vi "advance array manipulation part3.vi"() -> ()   [LabVIEW 2016]
panel:
  in  "Rotate index":i32
  out "Rotated Array":dbl[](array[numeric])
  in  "1D Input Array":dbl[](array[numeric])
  out "Reversed Array":dbl[](array[numeric])
  in  "1D Input Array":dbl[](array[numeric])
  out "Splited second Array":dbl[](array[numeric])
  out "Splited first Array":dbl[](array[numeric])
  in  "Split index":i32
  in  "1D Input Array":dbl[](array[numeric])
  out "Output index":i32
  in  "Search index":i32
  in  "Element":dbl
  in  "1D Input Array":dbl[](array[numeric])
  out "Output Array":dbl[](array[numeric])
  in  "1D Input Array":dbl[](array[numeric])
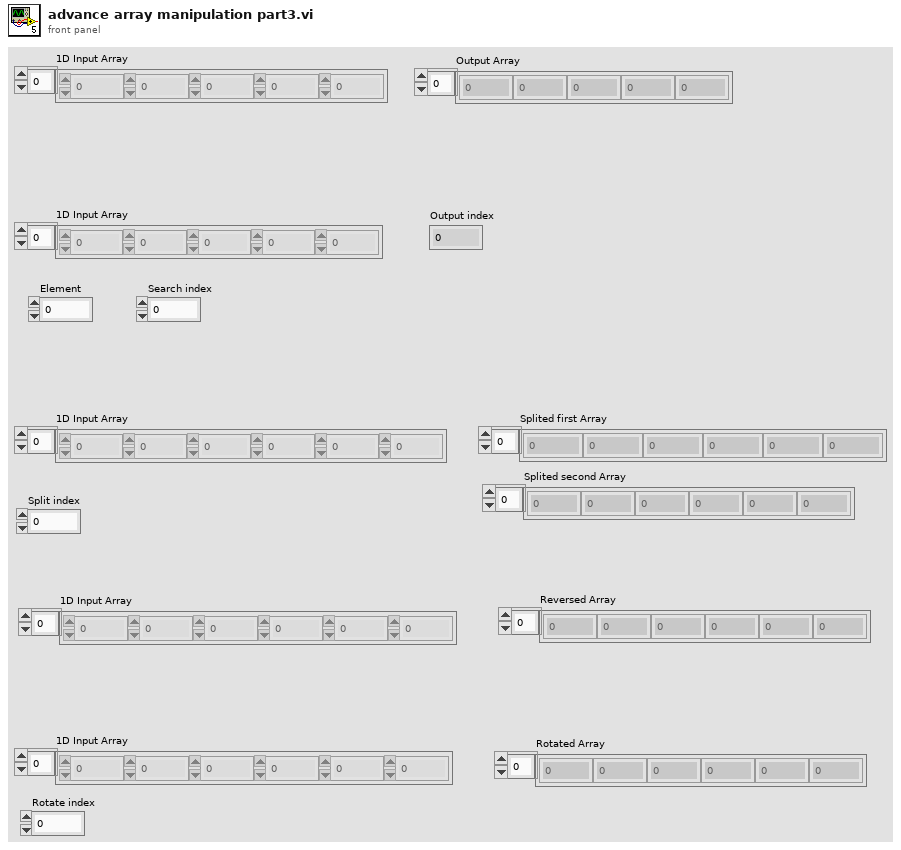
[diagram p1: front panel]
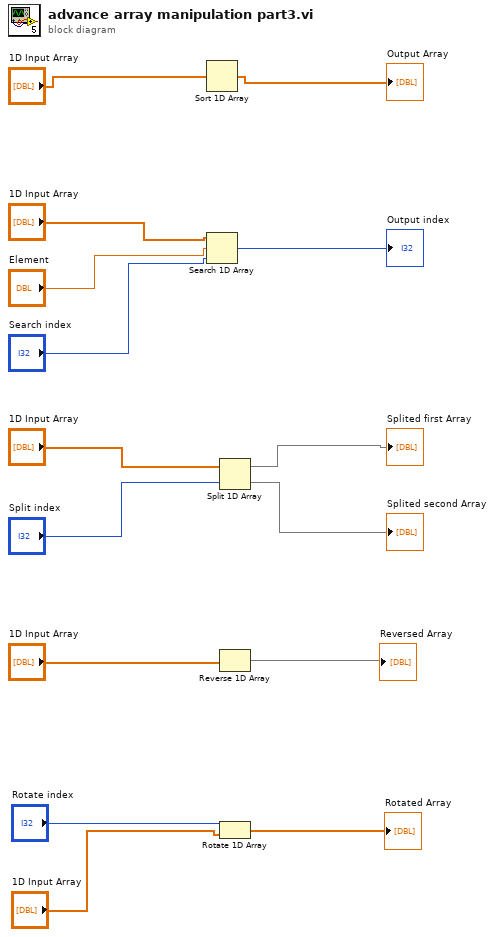
[diagram p0: block diagram]
diagram:
  n1 = Sort 1D Array(array="1D Input Array") -> (sorted array=→"Output Array":dbl[])
  n2 = Search 1D Array(1D array="1D Input Array", element="Element", start index (0)="Search index") -> (index of element=→"Output index":i32)
  n3 = Split 1D Array(array="1D Input Array", index="Split index") -> (first subarray=→"Splited first Array":dbl[], second subarray=→"Splited second Array":dbl[])
  n4 = Reverse 1D Array(array="1D Input Array") -> (reversed array=→"Reversed Array":dbl[])
  n5 = Rotate 1D Array(1:"1D Input Array", 2:"Rotate index") -> (0:→"Rotated Array":dbl[])
